vi "Interpret string.vi"(7 "Spreadsheet string":string) -> (2 "Time":string, 3 "Date":string, 4 "LineNumber":string, 6 "Qty of Optical Lines":string, 8 "OpticalLineNumber":string[](array[string]), 10 "Qty of FBG's":string[](array[string]), 13 "Peak Powers":string[][](array[string]), 14 "Peak Wavelengths":string[][](array[string]), 15 "System Status":string[][](array[string]))   [LabVIEW 2024]
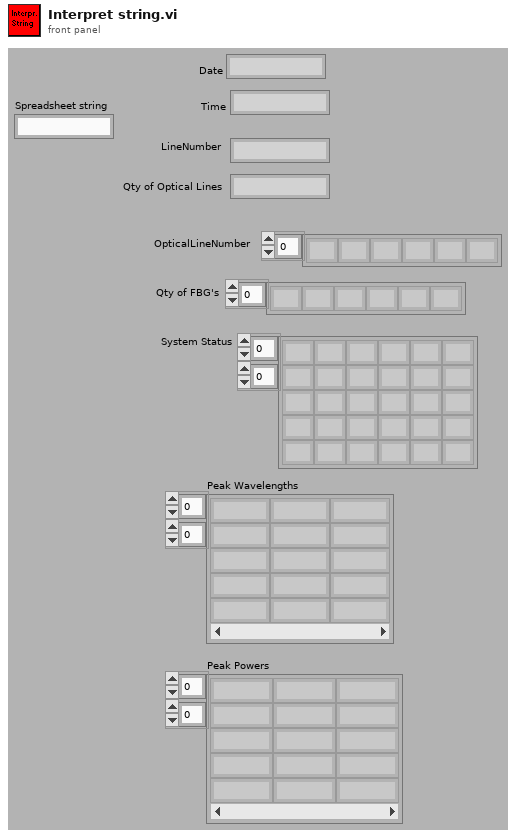
[diagram p1: front panel]
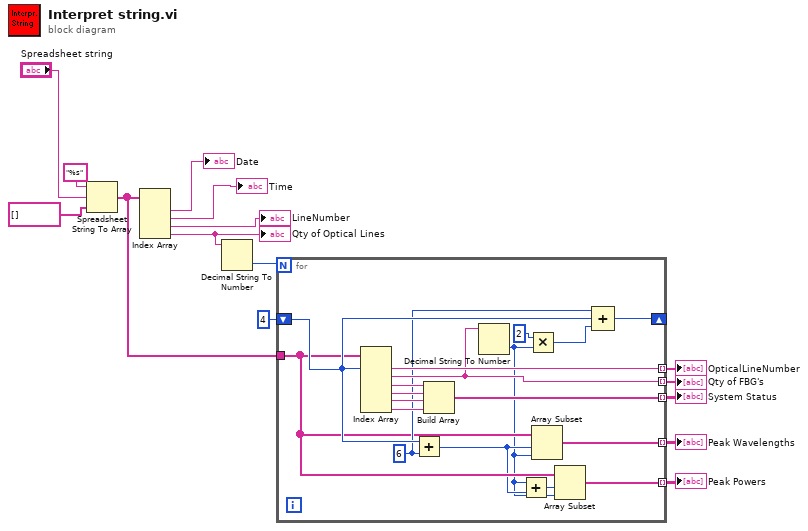
[diagram p0: block diagram]
diagram:
  n1 = Spreadsheet String To Array(format string="%s", spreadsheet string="Spreadsheet string", array type (2D Dbl)=string[] [] ("appended array")) -> (array=w9:string[])  [unwired: 1 in]
  n2 = Index Array(array=w9) -> (element #1=→"Date":string, element #2=→"Time":string, element #3=→"LineNumber":string, element #4=w3:string)  [unwired: 4 in]
  "Qty of Optical Lines" <- w3
  n3 = Decimal String To Number(string=w3) -> (number=w8:i32)  [unwired: 2 in, 1 out]
  n4 = for {
    N: w8 -> [_]
    tunnel: w9 -> [w21]
    shift-right: [w24] -> _
    shift-left: 4 -> [w23]
    tunnel: [w33] -> w11 mode=indexing
    tunnel: [w27] -> w12 mode=indexing
    tunnel: [w28] -> w13 mode=indexing
    tunnel: [w17] -> w14 mode=indexing
    tunnel: [w16] -> w15 mode=indexing
    w22 = 6 ("x")
    n5 = Index Array(array=w21, index #1=w23) -> (element #1=w33:string, element #2=w27:string, element #3=w32:string, element #4=w31:string, element #5=w30:string, element #6=w29:string)  [unwired: 5 in]
    n6 = Add(x=w23, y=w22) -> (x+y=w19:i32)
    n7 = Build Array(w32, w31, w30, w29) -> (w28:string[])
    n8 = Decimal String To Number(string=w27) -> (number=w18:i32)  [unwired: 2 in, 1 out]
    n9 = Add(x=w18, y=w19) -> (x+y=w20:i32)
    n10 = Multiply(x=2, y=w18) -> (x*y=w25:i32)
    n11 = Array Subset(array=w21, index=w19, length=w18) -> (w17:string[])
    n12 = Array Subset(array=w21, index=w20, length=w18) -> (w16:string[])
    n13 = Compound Arithmetic op=ADD(w22, w23, w25) -> (w24:i32)
  }
  "OpticalLineNumber" <- w11
  "Qty of FBG's" <- w12
  "System Status" <- w13
  "Peak Wavelengths" <- w14
  "Peak Powers" <- w15
